vi "Auto Shoot Using Dashboard Data.vi"(0 "Auto Preparation for Shooting":bool, 1 "Pilot X":dbl, 3 "Pilot Y":dbl, 4 "Elevation":dbl, 5 "Shoot Motors":dbl, 7 "Le Fire At Will":bool, 8 "Camera Centered?":bool, 9 "ReCenterize":bool, 10 "Stop Centerizing":bool, 11 "Set Point RPM":dbl, 13 "Fine Tune":bool, 14 "Stop Angle Adjust":bool, 15 "Angle Set Point":dbl, 16 "Cam offset - Delta X %":dbl, 17 "override \"Ready to Fire\"":bool) -> (21 "X Drive Arcade":dbl, 25 "Y Drive Arcade":dbl, 27 "Ready to Fire!":bool)   [LabVIEW 2012]
uses:
  Motors Values.vi
  BotStatus.vi
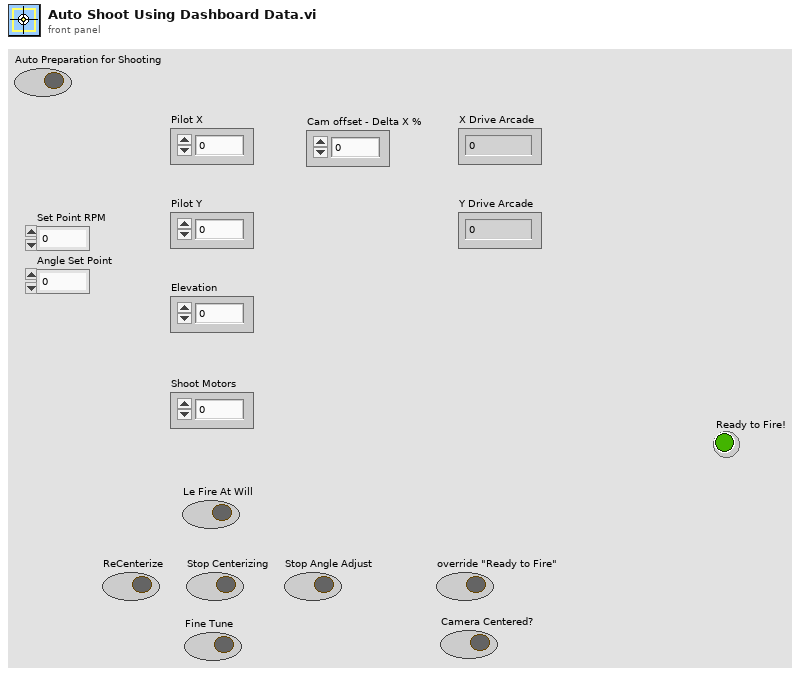
[diagram p1: front panel]
types:
  T1 = cluster{"Target Position X":dbl, "Target Position Y":dbl, "Target Found":bool}
  T2 = cluster{"Middle":bool, "InCannon":bool, "InFlipper":bool, "FlipperAtPlace":bool, "Bottom":bool, "FrisbeeDirection":bool}
  T3 = typedef "WPI_EncoderDevRef.ctl" = cluster{"DevStatus":errorcluster, "EncoderIndex":T4, "CounterIndex":T5, "DistancePerCount":dbl, "Decoding Type":T6}
  T4 = typedef "FPGA_EncoderIdx.ctl" = enum8{"Enc 0", "Enc 1", "Enc 2", "Enc 3", "Invalid"}
  T5 = typedef "FPGA_CounterCtrSystemIndex.ctl" = enum8{"Ctr 0", "Ctr 1", "Ctr 2", "Ctr 3", "Ctr 4", "Ctr 5", "Ctr 6", "Ctr 7", "Invalid"}
  T6 = typedef "WPI_EncoderType.ctl" = enum16{"1x", "2x", "4x"}
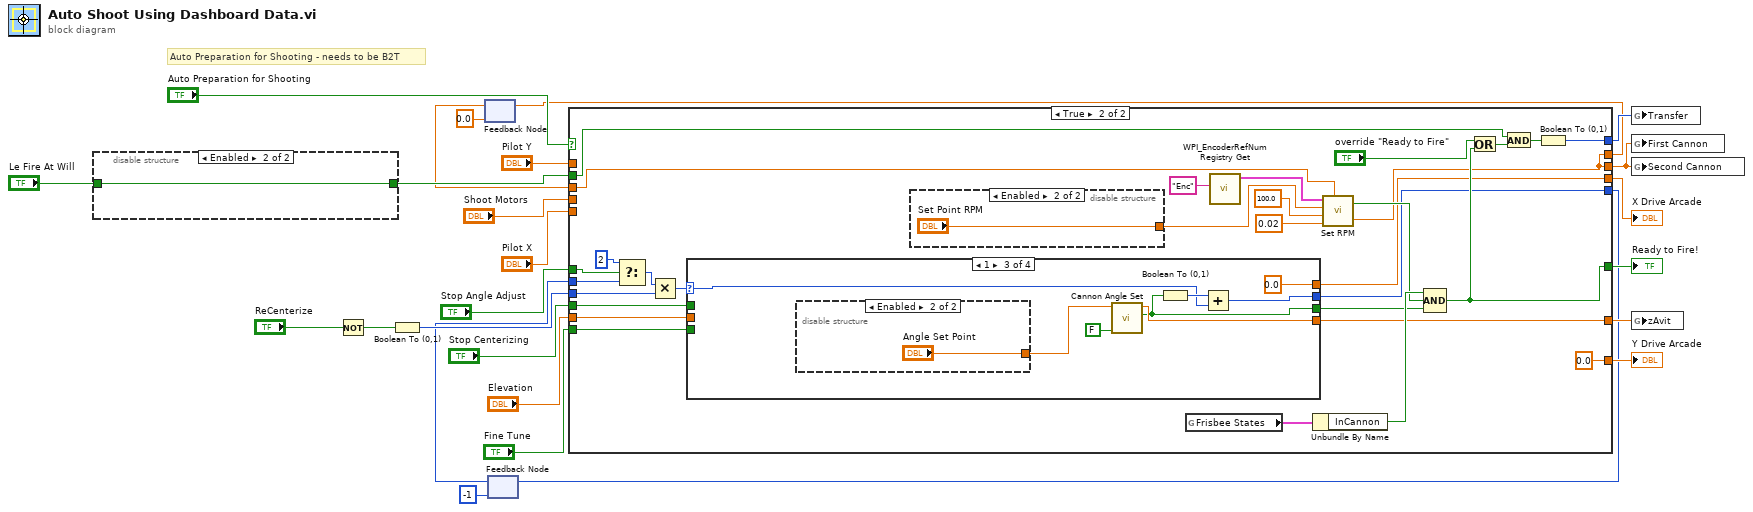
[diagram p0: block diagram]
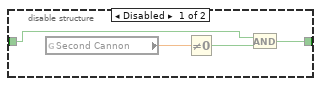
[diagram p2: hidden frame]
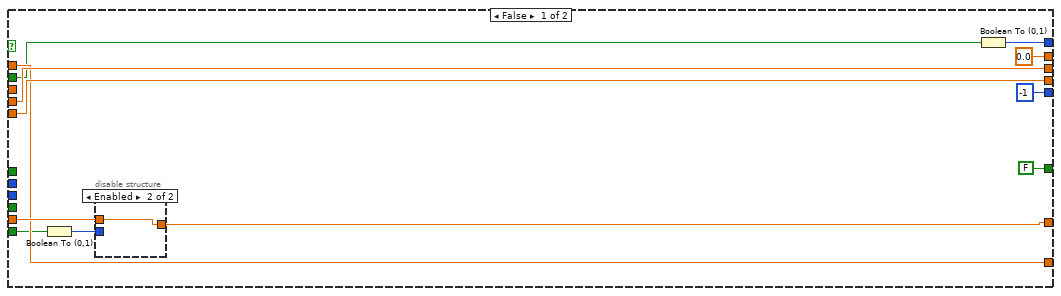
[diagram p3: hidden frame]
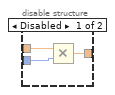
[diagram p4: hidden frame]
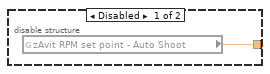
[diagram p5: hidden frame]
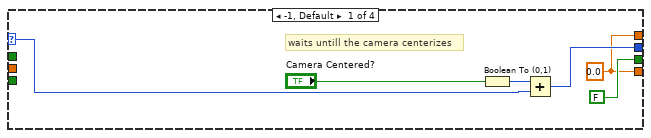
[diagram p6: hidden frame]
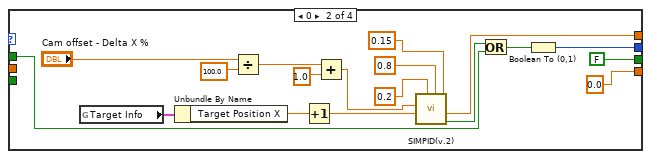
[diagram p7: hidden frame]
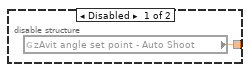
[diagram p8: hidden frame]
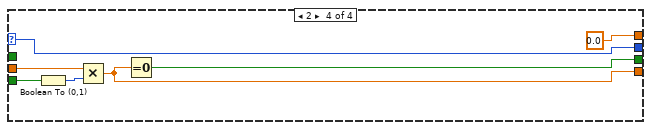
[diagram p9: hidden frame]
diagram:
  # "Auto Preparation for Shooting - needs to be B2T"
  n1 = disable-structure shown="Enabled" {
    disable-tunnel: "Le Fire At Will" -> [w27 w30]
    disable-tunnel: [w26 w30] -> w14
    frame Disabled {
      n2 = global read "Motors Values.vi" "Second Cannon"() -> (w29:dbl)
      n3 = Not Equal To 0?(x=w29) -> (x != 0?=w28:bool)
      n4 = And(x=w27, y=w28) -> (x .and. y?=w26:bool)
    }
    frame Enabled {
    }
  }
  n5 = Not(x="ReCenterize") -> (.not. x?=w10:bool)
  n6 = Boolean To (0,1)(Boolean=w10) -> (0, 1=w9:i16)
  n7 = feedback #1(0.0 ("Vbus Out")) -> (w3:dbl)
  n8 = feedback #2(-1) -> (w7:i32)
  n9 = case shown="True" "Auto Preparation for Shooting" {
    tunnel: [w37 w54] -> w22
    tunnel: [w42 w55] -> w23
    tunnel: "Pilot X" -> [w42 _]
    tunnel: "Elevation" -> [w41 w50]
    tunnel: w14 -> [w35 w71]
    tunnel: [w40 w74] -> w20
    tunnel: [w39 w48] -> w1
    tunnel: "Shoot Motors" -> [w39 _]
    tunnel: "Pilot Y" -> [w38 _]
    tunnel: [w38 0.0] -> w17
    tunnel: [FALSE w67] -> w16
    tunnel: "Fine Tune" -> [w33 w49]
    tunnel: "Stop Centerizing" -> [_ w51]
    tunnel: w9 -> [_ w68]
    tunnel: w7 -> [_ w64]
    tunnel: [-1 w56] -> w6
    tunnel: "Stop Angle Adjust" -> [_ w52]
    tunnel: [0.0 ("Vbus Out") w48] -> w4
    tunnel: w3 -> [_ w47]
    frame False {
      n10 = Boolean To (0,1)(Boolean=w33) -> (0, 1=w36:i16)
      n11 = disable-structure shown="Enabled" {
        disable-tunnel: w41 -> [w45 w46]
        disable-tunnel: [w44 w46] -> w37
        disable-tunnel: w36 -> [w43 _]
        frame Disabled {
          n12 = Multiply(x=w45, y=w43) -> (x*y=w44:dbl)
        }
        frame Enabled {
        }
      }
      n13 = Boolean To (0,1)(Boolean=w35) -> (0, 1=w40:i16)
    }
    frame True {
      n14 = Select(t=2, s=w52, f=w64) -> (s? t:f=w69:i32)
      n15 = Multiply(x=w69, y=w68) -> (x*y=w57:i32)
      n16 = case shown="1" w57 {
        selector: w57 -> [w82 _ w104 w115]
        tunnel: [w79 w95 0.0 ("Pilot X") 0.0 ("Pilot X")] -> w55
        tunnel: [w81 w94 w103 w115] -> w56
        tunnel: [w79 0.0 ("zAvit Vbus Out") w109 w116] -> w54
        tunnel: [FALSE ("On Target") FALSE ("On Target") w105 w117] -> w53
        tunnel: w51 -> [_ w85 _ _]
        tunnel: w50 -> [_ _ _ w118]
        tunnel: w49 -> [_ _ _ w113]
        frame -1, Default {
          w79 = 0.0 ("Pilot X")
          # "waits untill the camera centerizes"
          n17 = Boolean To (0,1)(Boolean="Camera Centered?") -> (0, 1=w83:i16)
          n18 = Add(x=w83, y=w82) -> (x+y=w81:i32)
        }
        frame 0 {
          n19 = global read "BotStatus.vi" "Target Info"() -> (w97:T1)
          n20 = Unbundle By Name(w97) -> ("Target Position X"=w96:dbl)
          n21 = Divide(x="Cam offset - Delta X %", y=100.0) -> (x/y=w89:dbl)
          n22 = Increment(x=w96) -> (x+1=w101:dbl)
          n23 = Add(x=w89, y=1.0 ("Set Point")) -> (x+y=w90:dbl)
          n24 = call "SIMPID(v.2).vi"("Range"=0.15, "upper limit"=0.8, "lower limit"=0.2, "Current Point"=w101, "Set Point"=w90) -> ("On Target"=w87:bool, "result"=w95:dbl)  [unwired: 5 in]
          n25 = Or(x=w87, y=w85) -> (x .or. y?=w86:bool)
          n26 = Boolean To (0,1)(Boolean=w86) -> (0, 1=w94:i16)
        }
        frame 1 {
          n27 = disable-structure shown="Enabled" {
            disable-tunnel: [w111 "Angle Set Point"] -> w110
            frame Disabled {
              n28 = global read "BotStatus.vi" "zAvit angle set point - Auto Shoot"() -> (w111:dbl)
            }
            frame Enabled {
            }
          }
          n29 = call "Cannon Angle Set.vi"("set angle 0 to be min angle"=FALSE, "Angle Set Point"=w110) -> ("On Target"=w105:bool, "zAvit Vbus Out"=w109:dbl)  [unwired: 8 in]
          n30 = Boolean To (0,1)(Boolean=w105) -> (0, 1=w106:i16)
          n31 = Add(x=w106, y=w104) -> (x+y=w103:i32)
        }
        frame 2 {
          n32 = Boolean To (0,1)(Boolean=w113) -> (0, 1=w119:i16)
          n33 = Multiply(x=w118, y=w119) -> (x*y=w116:dbl)
          n34 = Equal To 0?(x=w116) -> (x = 0?=w117:bool)
        }
      }
      n35 = disable-structure shown="Enabled" {
        disable-tunnel: [w77 "Set Point RPM"] -> w61
        frame Disabled {
          n36 = global read "BotStatus.vi" "zAvit RPM set point - Auto Shoot"() -> (w77:dbl)
        }
        frame Enabled {
        }
      }
      n37 = global read "BotStatus.vi" "Frisbee States"() -> (w76:T2)
      n38 = call <vilib>:"WPI_EncoderRefNum Registry Get.vi"("refnum name"="Enc") -> ("EncoderDevRef"=w62:T3)  [unwired: 9 in, 1 out]
      n39 = Unbundle By Name(w76) -> ("InCannon"=w75:bool)
      n40 = call "Set RPM.vi"("EncoderDevRef"=w62, "Set Point RPM"=w61, "Range RPM"=100.0, "Gain Vbus"=0.02, "Previous Vbus"=w47) -> ("READY!"=w58:bool, "Vbus Out"=w48:dbl)
      n41 = Compound Arithmetic op=AND(w75, w58, w53) -> (w67:bool)
      n42 = Or(x="override \"Ready to Fire\"", y=w67) -> (x .or. y?=w65:bool)
      n43 = And(x=w71, y=w65) -> (x .and. y?=w72:bool)
      n44 = Boolean To (0,1)(Boolean=w72) -> (0, 1=w74:i16)
    }
  }
  "X Drive Arcade" <- w23
  "Y Drive Arcade" <- w17
  "Ready to Fire!" <- w16
  n45 = feedback-in #1(w4) -> ()
  n46 = feedback-in #2(w6) -> ()
  n47 = global write "Motors Values.vi" "Transfer"(w20) -> ()
  n48 = global write "Motors Values.vi" "First Cannon"(w1) -> ()
  n49 = global write "Motors Values.vi" "Second Cannon"(w1) -> ()
  n50 = global write "Motors Values.vi" "zAvit"(w22) -> ()
